vi "test_mode_control.vi"(2 "values in":cluster{"test_mode":string}) -> (6 "test_mode":string)   [LabVIEW 2015]
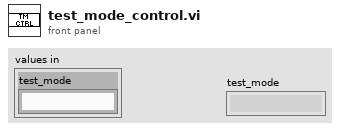
[diagram p1: front panel]
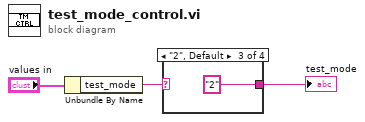
[diagram p0: block diagram]
diagram:
  n1 = Unbundle By Name("values in") -> ("test_mode"=w2:string)
  n2 = case shown="\"2\", Default" w2 {
    selector: w2 -> [w4 w5 _ w7]
    tunnel: [w4 w5 "2" w7] -> w1
    frame "0" {
    }
    frame "1" {
    }
    frame "2", Default {
    }
    frame "3" {
    }
  }
  "test_mode" <- w1
